vi "Read Flow Control.vi"(8 "error in (no error)":errorcluster, 11 "serial slave in":refnum<class "Serial Slave.lvclass">) -> (0 "error out":errorcluster, 2 "flow control":u16(ring) items=["None", "XON/XOFF", "RTS/CTS", "XON/XOFF & RTS/CTS", "DTR/DSR", "XON/XOFF & DTR/DSR"], 3 "serial slave out":refnum<class "Serial Slave.lvclass">)   [LabVIEW 2018, in "SubVIs.lvlib" / "Serial Slave.lvclass"]
uses:
  Serial Slave.lvclass
  Serial Slave.lvclass/Serial Slave.ctl
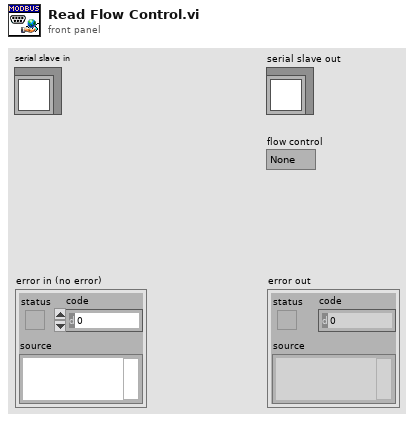
[diagram p1: front panel]
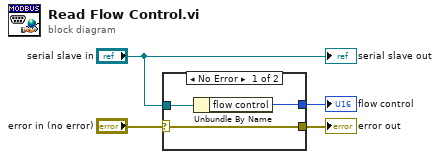
[diagram p0: block diagram]
diagram:
  n1 = case shown="No Error" "error in (no error)" {
    selector: "error in (no error)" -> [w5 w8]
    tunnel: "serial slave in" -> [w7 _]
    tunnel: [w6 _] -> w3
    tunnel: [w5 w8] -> w1
    frame No Error {
      n2 = Unbundle By Name(w7) -> ("flow control"=w6:u16)
    }
    frame Error {
    }
  }
  "error out" <- w1
  "flow control" <- w3
  "serial slave out" <- "serial slave in"
